vi "Autonomous Independent.vi"() -> ()   [LabVIEW 2013]
doc: "This VI is called when autonomous begins, and will automatically be terminated when autonomous ends. You can carry out timed or sensor driven robot movement independently without needing to return to the caller."
uses:
  <vilib>/Rock Robotics/WPI/Solenoid/WPI_SolenoidValue.ctl
  Robot Global Data.vi
  Systems/Sensors/Sensors Global Values.vi
panel:
  in  "drive forward to collect ball time":u32
  in  "Distance wanted (ft)":dbl=6.0 format="%#_13g"
  # "Be sure to right-click and choose Data Operations>>Make Current Value default if you want to save the array values with the VI"
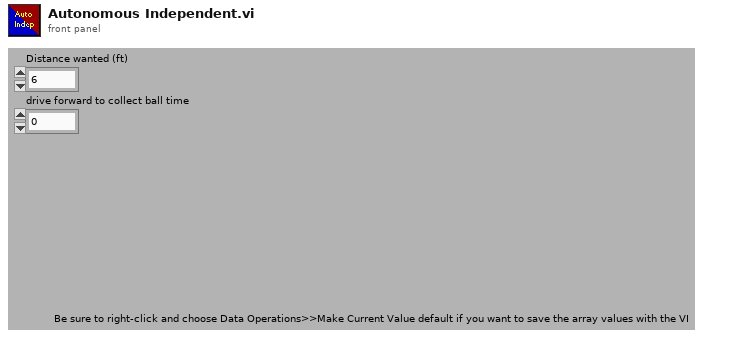
[diagram p1: front panel]
types:
  T1 = typedef "WPI_SolenoidValue.ctl" = enum16{"Off", "On", "Forward", "Reverse"}
  T2 = cluster{"Camera Sonar":dbl, "Front Right Sonar":dbl, "Front Left Sonar":dbl, "Rear Sonar":dbl}
  T3 = typedef "WPI_ServoDeviceRef.ctl" = cluster{"DeviceStatus":errorcluster, "Digital Module":T4, "PWM Channel":T5, "DeadBand":T6}
  T4 = typedef "FPGA_TypedefDigitalModule.ctl" = enum16{"Digital Module 1", "Digital Module 2"}
  T5 = typedef "FPGA_DIOPWMChannel.ctl" = enum8{"PWM 1", "PWM 2", "PWM 3", "PWM 4", "PWM 5", "PWM 6", "PWM 7", "PWM 8", "PWM 9", "PWM 10", "Invalid"}
  T6 = typedef "WPI_PWMDeadband.ctl" = cluster{"Name":string, "maxPositivePwm":i32, "minPositivePwm":i32, "centerPwm":i32, "maxNegativePwm":i32, "minNegativePwm":i32, "angularRange":u16}
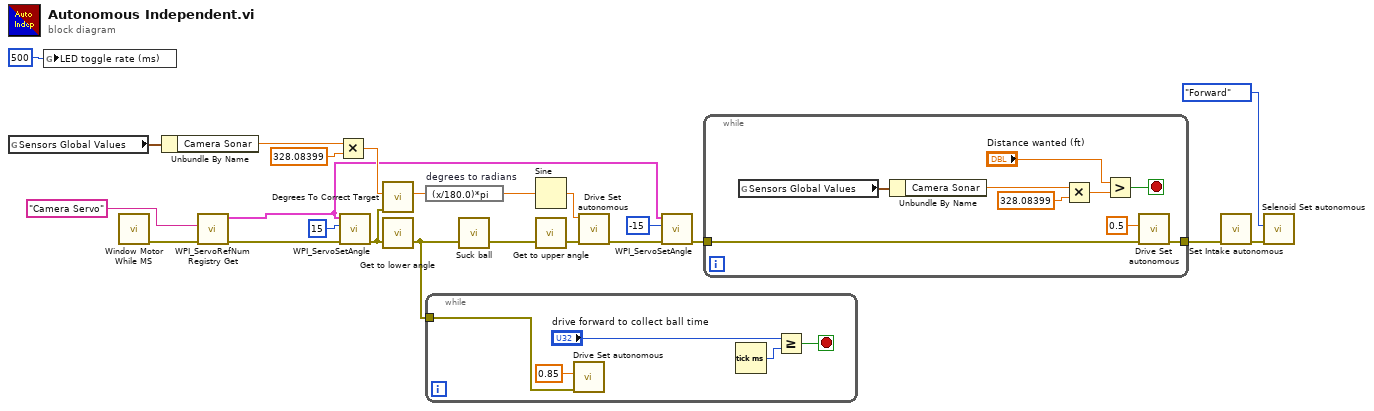
[diagram p0: block diagram]
diagram:
  n1 = global read "Sensors Global Values.vi" "Sensors Global Values"() -> (w22:T2)
  n2 = global write "Robot Global Data.vi" "LED toggle rate (ms)"(u32 500 ("LED ms toggle rate")) -> ()
  n3 = call "Window Motor While MS.vi"() -> ("error out"=w7:errorcluster)  [unwired: 11 in]
  n4 = Unbundle By Name(w22) -> ("Camera Sonar"=w16:dbl)
  n5 = call <vilib>:"WPI_ServoRefNum Registry Get.vi"("error in (no error)"=w7, "refnum name"="Camera Servo") -> ("error out"=w6:errorcluster, "ServoDeviceRef"=w11:T3)  [unwired: 8 in]
  n6 = Multiply(x=w16, y=328.08399) -> (x*y=w15:dbl)
  n7 = call <vilib>:"WPI_ServoSetAngle.vi"("error in (no error)"=w6, "Angle"=15, "ServoDeviceRef"=w11) -> ("error out"=w5:errorcluster)  [unwired: 7 in, 1 out]
  n8 = call "Degrees To Correct Target.vi"("error in"=w5, "Distance to Wall (ft)"=w15) -> ("Degrees"=w20:dbl)  [unwired: 8 in, 1 out]
  n9 = call "Get to lower angle.vi"("error in (no error)"=w5) -> ("error out"=w1:errorcluster)  [unwired: 2 in]
  n10 = expression code="(x/180.0)*pi" "degrees to radians"(w20) -> (w21:dbl)
  n11 = while {
    tunnel: w1 -> [w24]
    stop <- w26 stop-if-true
    n12 = call "Drive Set autonomous.vi"("error in (no error)"=w24, "Y value"=0.85) -> ()  [unwired: 9 in, 1 out]
    n13 = Tick Count (ms)() -> (millisecond timer value=w28:u32)
    n14 = Greater Or Equal?(x="drive forward to collect ball time", y=w28) -> (x >= y?=w26:bool)
  }
  n15 = call "Suck ball.vi"("error in (no error)"=w1) -> ("error out"=w14:errorcluster)  [unwired: 2 in]
  n16 = Sine(x=w21) -> (sin(x)=w19:dbl)
  n17 = call "Get to upper angle.vi"("error in (no error)"=w14) -> ("error out"=w13:errorcluster)  [unwired: 2 in]
  n18 = call "Drive Set autonomous.vi"("error in (no error)"=w13, "X value"=w19) -> ("error out (no error)"=w4:errorcluster)  [unwired: 9 in]
  n19 = call <vilib>:"WPI_ServoSetAngle.vi"("error in (no error)"=w4, "Angle"=-15, "ServoDeviceRef"=w11) -> ("error out"=w3:errorcluster)  [unwired: 7 in, 1 out]
  n20 = while {
    tunnel: w3 -> [w30]
    tunnel: [w29] -> w2
    stop <- w36 stop-if-true
    n21 = global read "Sensors Global Values.vi" "Sensors Global Values"() -> (w33:T2)
    n22 = Unbundle By Name(w33) -> ("Camera Sonar"=w32:dbl)
    n23 = Multiply(x=w32, y=328.08399) -> (x*y=w34:dbl)
    n24 = Greater?(x="Distance wanted (ft)", y=w34) -> (0:w36:bool)
    n25 = call "Drive Set autonomous.vi"("error in (no error)"=w30, "Y value"=0.5 ("Y axis value")) -> ("error out (no error)"=w29:errorcluster)  [unwired: 9 in]
  }
  n26 = call "Set Intake autonomous.vi"("error in (no error)"=w2) -> ("error out"=w12:errorcluster)  [unwired: 10 in]
  n27 = call "Selenoid Set autonomous.vi"("error in (no error)"=w12, "Value"=WPI_SolenoidValue."Forward") -> ()  [unwired: 9 in, 1 out]
